vi "Publish (async).vi"(4 "ArgumentsKw":string, 6 "Arguments":variant[](array[variant]), 7 "Request Ack.":bool, 8 "Error in":errorcluster, 9 "Topic":string, 11 "WAMP Client in":refnum<class "WAMP Client.lvclass">) -> (0 "Error cout":errorcluster, 1 "Publish Results Event":refnum<user-event>, 3 "WAMP Client out":refnum<class "WAMP Client.lvclass">)   [LabVIEW 2020, in "wamplv.lvlib" / "WAMP Client.lvclass"]
uses:
  WAMP Client.lvclass
  TypeDef/PUBLISH result2.ctl
  TypeDefs/Combined error.ctl
  TypeDefs/WAMP error.ctl
  TypeDef/Internal Message Type.ctl
  TypeDef/PUBLISH Request Data.ctl
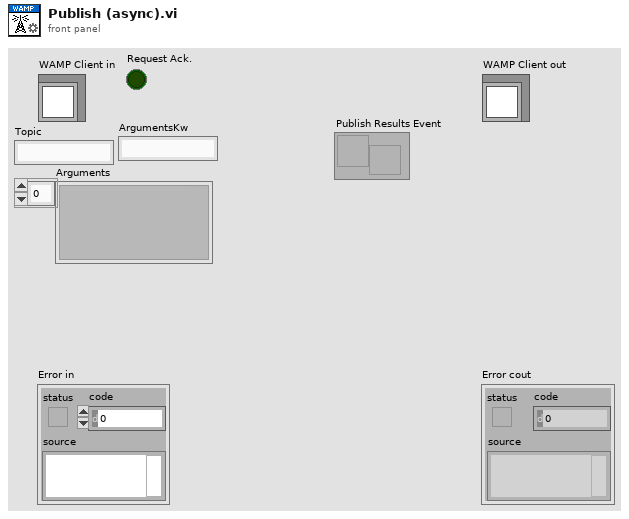
[diagram p1: front panel]
types:
  T1 = typedef "wamplv.lvlib/WAMP Client.lvclass/PUBLISH Request Data.ctl" = cluster{"Topic URI":string, "Arguments":variant[], "ArgumentsKw":string, "Publish Result Event":refnum<user-event>, "Request Ackoweldegemtn":bool}
  T2 = typedef "wamplv.lvlib/WAMP Client.lvclass/PUBLISH result2.ctl" = cluster{"Publish Request ID":u64, "Publication ID":u64, "Success?":bool, "Combined Error":T3}
  T3 = typedef "wamplv.lvlib/WAMP Client.lvclass/Combined error.ctl" = cluster{"Error?":bool, "WAMP Error":T4, "Error":errorcluster}
  T4 = typedef "wamplv.lvlib/WAMP Client.lvclass/WAMP error.ctl" = cluster{"Details":string, "ArgumentKw Payload":string, "Error?":bool, "Error URI":string, "Arguments Payload":string[]}
  T5 = typedef "wamplv.lvlib/WAMP Client.lvclass/Internal Message Type.ctl" = enum16{"Subscribe", "Handle Subscribed", "Handle Event", "Unsubscribe", "Handle Unsubscribed", "Publish", "Handled Published", "Goodbye", "Handle Goodbye", "Call", "Handle Result", "Register", "Handle Registered", "Unregister", "Handle Unregistered", "Handle Invocation", "Yield", "Error"}
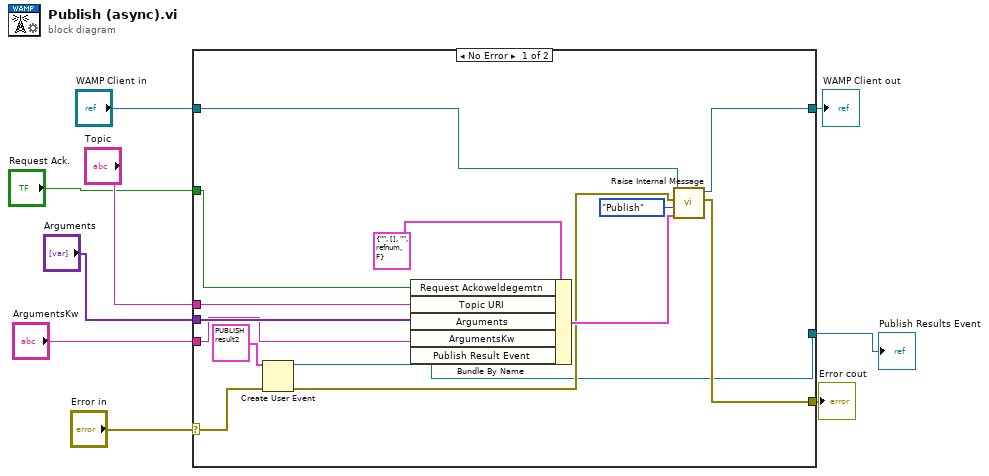
[diagram p0: block diagram]
diagram:
  n1 = case shown="No Error" "Error in" {
    selector: "Error in" -> [w17 w25]
    tunnel: [w15 w25] -> w8
    tunnel: [w14 w24] -> w6
    tunnel: "WAMP Client in" -> [w23 w24]
    tunnel: "Topic" -> [w21 _]
    tunnel: "Arguments" -> [w13 _]
    tunnel: "ArgumentsKw" -> [w12 _]
    tunnel: [w11 _] -> w2
    tunnel: "Request Ack." -> [w10 _]
    frame No Error {
      n2 = Create User Event(user event datatype=T2 {"Publish Request ID"=0, "Publication ID"=0, "Success?"=FALSE, "Combined Error"={"Error?"=FALSE, "WAMP Error"={"Details"="", "ArgumentKw Payload"="{}", "Error?"=FALSE, "Error URI"="", "Arguments Payload"=[]}, "Error"={"status"=FALSE, "code"=0, "source"=""}}} ("Cluster"), error in=w17) -> (user event=w11:refnum<user-event>, error out=w16:errorcluster)
      n3 = Bundle By Name(cluster=T1 {"Topic URI"="", "Arguments"=[], "ArgumentsKw"="", "Publish Result Event"=refnum, "Request Ackoweldegemtn"=FALSE} ("Cluster"), "Request Ackoweldegemtn"=w10, "Topic URI"=w21, "Arguments"=w13, "ArgumentsKw"=w12, "Publish Result Event"=w11) -> (w22:T1)
      n4 = call-dynamic "Raise Internal Message.vi"("Variant"=w22, "Internal Message Type"=Internal_Message_Type."Publish", "error in (no error)"=w16, "WAMP Client in"=w23) -> ("error out"=w15:errorcluster, "WAMP Client out"=w14:refnum<class "WAMP Client.lvclass">)  [unwired: 6 in]
    }
    frame Error {
    }
  }
  "Error cout" <- w8
  "WAMP Client out" <- w6
  "Publish Results Event" <- w2
